vi "init.vi"(0 "StartTestScenarioCommand in":refnum<class "StartTestScenarioCommand.lvclass">, 5 "Serial Number":string, 7 "Operator":string, 9 "Comments":string, 11 "error in (no error)":errorcluster) -> (4 "StartTestScenarioCommand out":refnum<class "StartTestScenarioCommand.lvclass">, 15 "error out":errorcluster)   [LabVIEW 2015, in "StartTestScenarioCommand.lvclass"]
uses:
  StartTestScenarioCommand.lvclass
  StartTestScenarioCommand.lvclass/StartTestScenarioCommand.ctl
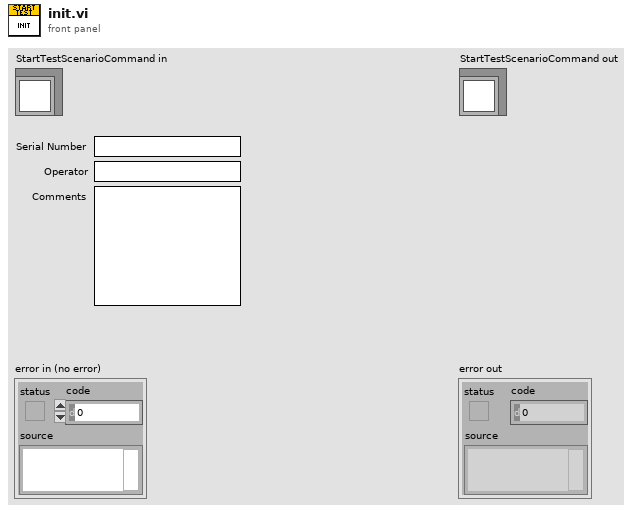
[diagram p1: front panel]
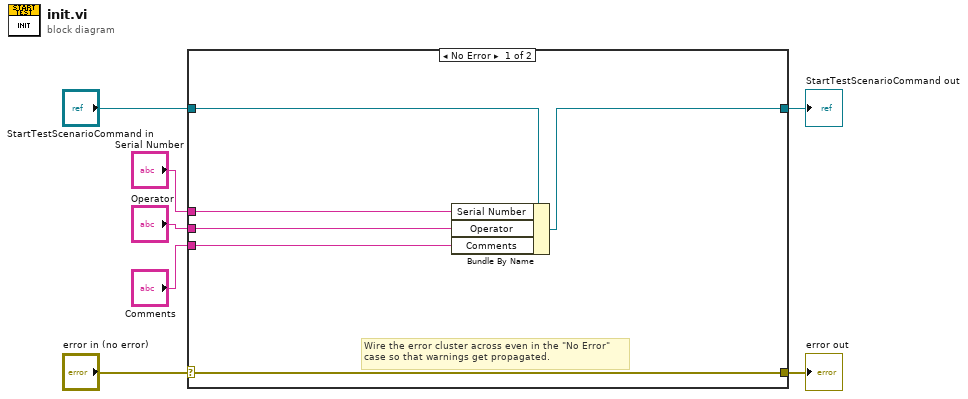
[diagram p0: block diagram]
diagram:
  n1 = case shown="No Error" "error in (no error)" {
    selector: "error in (no error)" -> [w13 w15]
    tunnel: [w13 w15] -> w6
    tunnel: [w11 w14] -> w4
    tunnel: "StartTestScenarioCommand in" -> [w12 w14]
    tunnel: "Serial Number" -> [w10 _]
    tunnel: "Operator" -> [w9 _]
    tunnel: "Comments" -> [w8 _]
    frame No Error {
      # "Wire the error cluster across even in the \"No Error\"\ncase so that warnings get propagated."
      n2 = Bundle By Name(cluster=w12, "Serial Number"=w10, "Operator"=w9, "Comments"=w8) -> (w11:refnum<class "StartTestScenarioCommand.lvclass">)
    }
    frame Error {
    }
  }
  "error out" <- w6
  "StartTestScenarioCommand out" <- w4
